vi "5.10 Plotting Function for MicroAlg1.vi"(0 "Image Dst Out":T2, 1 "Line Definition":T1, 2 "Color":u32(colorbox), 3 "Group":string, 4 "Width":u32=3) -> (5 "Image Out":T2)   [LabVIEW 2010]
uses:
  <vilib>/vision/Image Controls.llb/IMAQ Image.ctl
  6-OCU Neurons/6.10 Occipital Neurons/6.10.1 LineDef.ctl
panel:
  out "Mean":cluster{"X":dbl, "Y":dbl}
  out "Algorithm out":T2(plugin-control)
  # "X"
  # "Y"
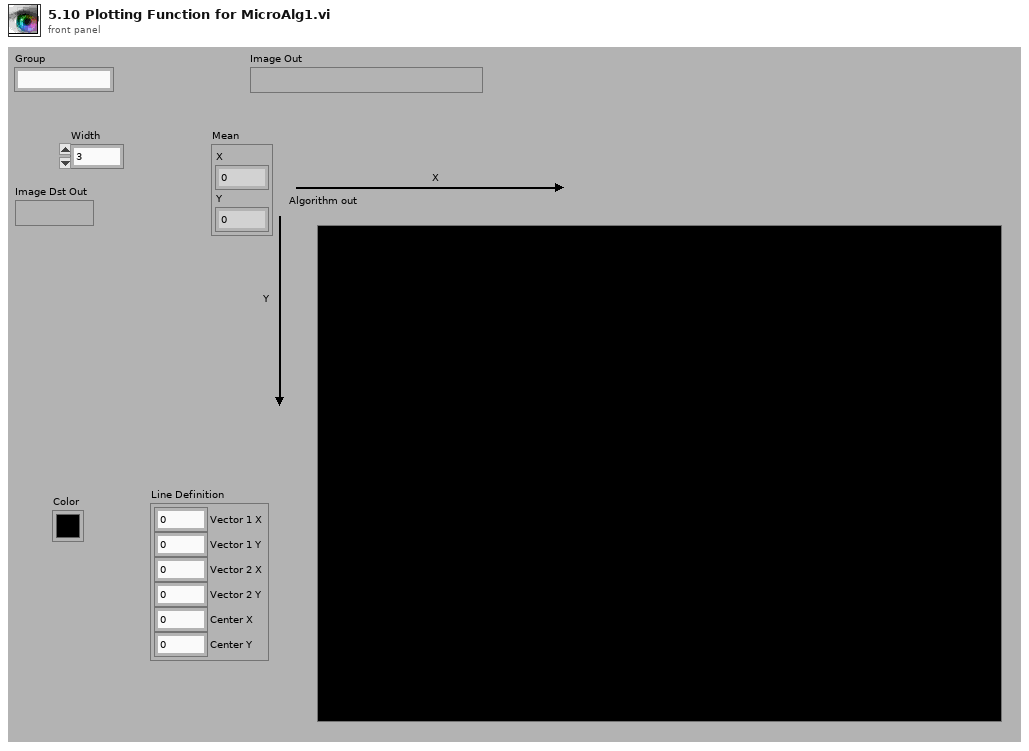
[diagram p1: front panel]
types:
  T1 = typedef "6.10.1 LineDef.ctl" = cluster{"Vector 1 X":dbl, "Vector 1 Y":dbl, "Vector 2 X":dbl, "Vector 2 Y":dbl, "Center X":dbl, "Center Y":dbl}
  T2 = typedef "IMAQ Image.ctl" = refnum<image>
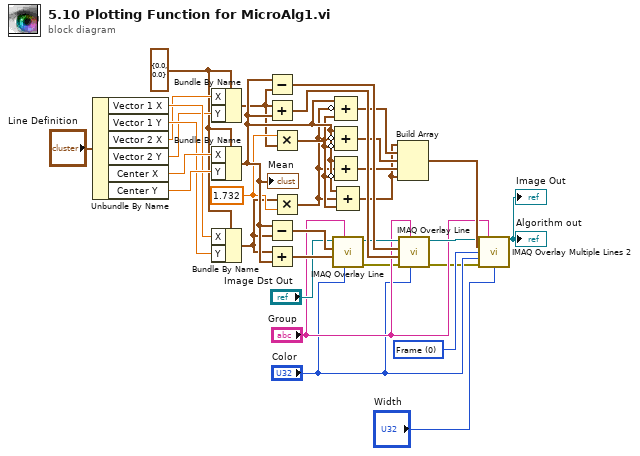
[diagram p0: block diagram]
diagram:
  w3 = 1.732
  w19 = u32 0 items=["Frame", "Fill"] ("Drawing Mode (Frame)")
  w20 = cluster{"X":dbl, "Y":dbl} {"X"=0.0, "Y"=0.0} ("Start Point")
  n1 = Unbundle By Name("Line Definition") -> ("Vector 1 X"=w24:dbl, "Vector 1 Y"=w23:dbl, "Vector 2 X"=w22:dbl, "Vector 2 Y"=w21:dbl, "Center X"=w25:dbl, "Center Y"=w26:dbl)
  n2 = Bundle By Name(cluster=w20, "X"=w22, "Y"=w21) -> (w2:cluster{"X":dbl, "Y":dbl})
  n3 = Bundle By Name(cluster=w20, "X"=w25, "Y"=w26) -> (w6:cluster{"X":dbl, "Y":dbl})
  "Mean" <- w6
  n4 = Bundle By Name(cluster=w20, "X"=w24, "Y"=w23) -> (w1:cluster{"X":dbl, "Y":dbl})
  n5 = Subtract(x=w6, y=w2) -> (x-y=w32:cluster{"X":dbl, "Y":dbl})
  n6 = Add(x=w2, y=w6) -> (x+y=w33:cluster{"X":dbl, "Y":dbl})
  n7 = Subtract(x=w6, y=w1) -> (x-y=w30:cluster{"X":dbl, "Y":dbl})
  n8 = Add(x=w1, y=w6) -> (x+y=w31:cluster{"X":dbl, "Y":dbl})
  n9 = Multiply(x=w3, y=w2) -> (x*y=w5:cluster{"X":dbl, "Y":dbl})
  n10 = Multiply(x=w1, y=w3) -> (x*y=w4:cluster{"X":dbl, "Y":dbl})
  n11 = call "IMAQ Overlay Line"("Color"="Color", "Group"="Group", "End Point"=w31, "Start Point"=w30, "Image"="Image Dst Out") -> ("error out"=w9:errorcluster, "Image Out"=w29:T2)  [unwired: 5 in]
  n12 = Compound Arithmetic op=ADD(w6, invert w4, w5) -> (w18:cluster{"X":dbl, "Y":dbl})
  n13 = Compound Arithmetic op=ADD(w6, invert w4, invert w5) -> (w17:cluster{"X":dbl, "Y":dbl})
  n14 = Compound Arithmetic op=ADD(w6, w4, invert w5) -> (w16:cluster{"X":dbl, "Y":dbl})
  n15 = Compound Arithmetic op=ADD(w6, w4, w5) -> (w7:cluster{"X":dbl, "Y":dbl})
  n16 = Build Array(w7, w18, w17, w16, w7) -> (w15:cluster{"X":dbl, "Y":dbl}[])
  n17 = call "IMAQ Overlay Line"("Color"="Color", "Group"="Group", "error in (no error)"=w9, "End Point"=w33, "Start Point"=w32, "Image"=w29) -> ("error out"=w10:errorcluster, "Image Out"=w14:T2)  [unwired: 4 in]
  n18 = call "IMAQ Overlay Multiple Lines 2"("Image"=w14, "Group"="Group", "Line End Points"=w15, "Drawing Mode (Frame)"=w19, "Color"="Color", "error in (no error)"=w10, "Width"="Width") -> ("Image Out"=→"Image Out" →"Algorithm out":T2)  [unwired: 7 in, 1 out]
